vi "trace.calling_method.vi"() -> (2 "Calling Method Name":string)   [LabVIEW 2020, in "Nominal Client.lvclass"]
uses:
  Nominal Client.lvclass
  Nominal Client.lvclass/Nominal Client.ctl
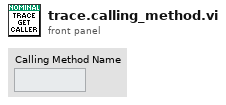
[diagram p1: front panel]
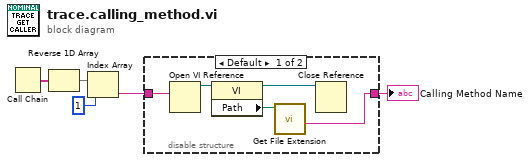
[diagram p0: block diagram]
diagram:
  n1 = Call Chain() -> (call chain=w3:string[])
  n2 = Reverse 1D Array(array=w3) -> (reversed array=w4:string[])
  n3 = Index Array(array=w4, index=1) -> (element=w2:string)
  n4 = disable-structure shown="Default" {
    disable-tunnel: w2 -> [w8 w11]
    disable-tunnel: [w6 w11] -> w1
    frame condition #0 (active) {
      n5 = Open VI Reference(vi path=w8) -> (vi reference=w9:refnum<vi>)  [unwired: 5 in, 1 out]
      n6 = property class="VI"(reference=w9) -> (reference out=w10:refnum<vi>, "Path"=w7:path)  [unwired: 1 in, 1 out]
      n7 = call <vilib>:"Get File Extension.vi"("file"=w7) -> ("filename without extension"=w6:string)  [unwired: 6 in, 4 out]
      n8 = Close Reference(reference=w10) -> ()  [unwired: 1 in, 1 out]
    }
    frame condition #1 {
    }
  }
  "Calling Method Name" <- w1
